vi "Write to File.vi"(7 "Channel Direction":string, 8 "error in (no error)":errorcluster, 10 "Channels":refnum<class "Channel.lvclass">[](array[class]), 11 "ConfigFile in":refnum<class "ConfigFile.lvclass">) -> (0 "error out":errorcluster, 3 "ConfigFile out":refnum<class "ConfigFile.lvclass">)   [LabVIEW 2020, in "ImportExport.lvlib" / "ConfigFile.lvclass"]
uses:
  ConfigFile.lvclass
  built/windows/Channel.lvlibp/Channel.lvclass
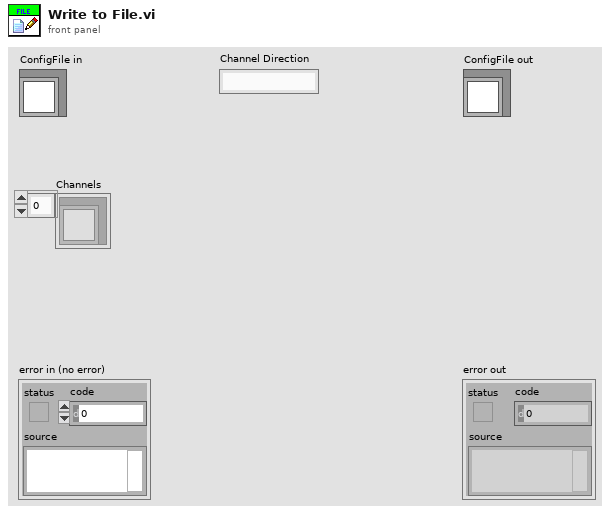
[diagram p1: front panel]
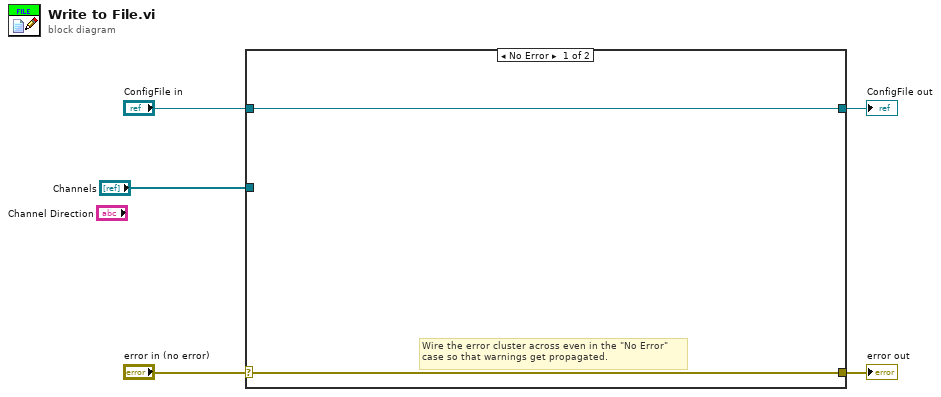
[diagram p0: block diagram]
diagram:
  n1 = case shown="No Error" "error in (no error)" {
    selector: "error in (no error)" -> [w6 w9]
    tunnel: [w6 w9] -> w4
    tunnel: [w7 w8] -> w2
    tunnel: "ConfigFile in" -> [w7 w8]
    tunnel: "Channels" -> [_ _]
    frame No Error {
      # "Wire the error cluster across even in the \"No Error\"\ncase so that warnings get propagated."
    }
    frame Error {
    }
  }
  "error out" <- w4
  "ConfigFile out" <- w2
